vi "Get Color.vi"() -> (0 "Matched Color Name":string)   [LabVIEW 2019]
uses:
  Robot Global Data.vi
panel:
  out "Measured Color":cluster{"R":dbl, "G":dbl, "B":dbl}
  in  "Blue Calibration":cluster{"R":dbl, "G":dbl, "B":dbl}={"R"=0.143, "G"=0.427, "B"=0.429}
  in  "Green Calibration":cluster{"R":dbl, "G":dbl, "B":dbl}={"R"=0.197, "G"=0.561, "B"=0.24}
  in  "Red Calibration":cluster{"R":dbl, "G":dbl, "B":dbl}={"R"=0.561, "G"=0.323, "B"=0.114}
  in  "Yellow Calibration":cluster{"R":dbl, "G":dbl, "B":dbl}={"R"=0.361, "G"=0.524, "B"=0.113}
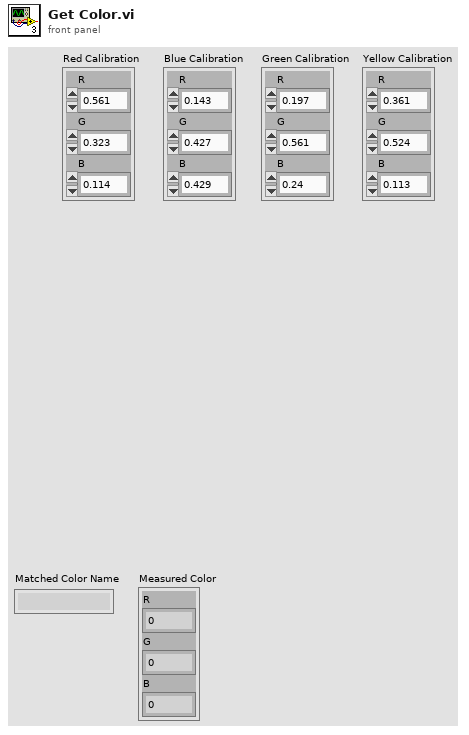
[diagram p1: front panel]
types:
  T1 = typedef "Color Sensor V3 DevRef.ctl" = cluster{"I2CDevRef":T2}
  T2 = typedef "WPI_I2CDevRef.ctl" = cluster{"DevStatus":errorcluster, "Device Address":u8, "Handle":i32, "I2C Bus":T3}
  T3 = typedef "i2c_bus.ctl" = enum16{"I2C On-Board", "I2C MXP", "Invalid"}
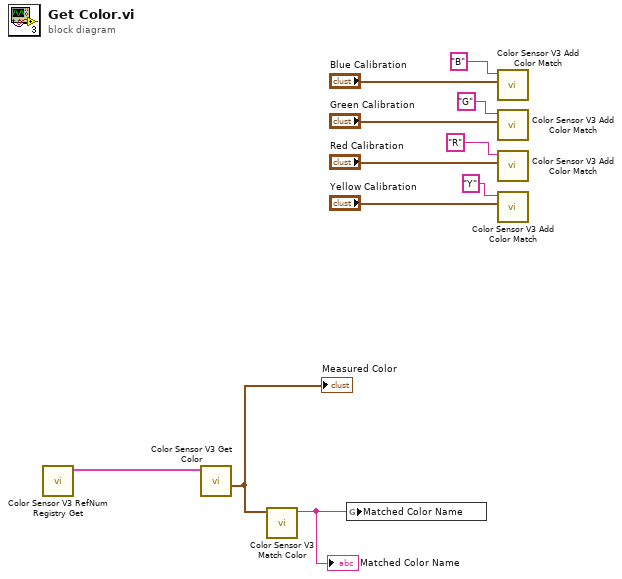
[diagram p0: block diagram]
diagram:
  n1 = call <vilib>:"Color Sensor V3 RefNum Registry Get.vi"() -> ("ColorSensorDevRef"=w2:T1)  [unwired: 10 in, 1 out]
  n2 = call <vilib>:"Color Sensor V3 Get Color.vi"("ColorSensorDevRef"=w2) -> ("Normalized Color"=w3:cluster{"R":dbl, "G":dbl, "B":dbl})  [unwired: 7 in, 3 out]
  "Measured Color" <- w3
  n3 = call <vilib>:"Color Sensor V3 Match Color.vi"("Measured Color"=w3) -> ("Matched Color Name"=w1:string)  [unwired: 8 in, 2 out]
  "Matched Color Name" <- w1
  n4 = global write "Robot Global Data.vi" "Matched Color Name"(w1) -> ()
  n5 = call <vilib>:"Color Sensor V3 Add Color Match.vi"("Color"="Blue Calibration", "Name"="B") -> ()  [unwired: 10 in]
  n6 = call <vilib>:"Color Sensor V3 Add Color Match.vi"("Color"="Green Calibration", "Name"="G") -> ()  [unwired: 10 in]
  n7 = call <vilib>:"Color Sensor V3 Add Color Match.vi"("Color"="Red Calibration", "Name"="R") -> ()  [unwired: 10 in]
  n8 = call <vilib>:"Color Sensor V3 Add Color Match.vi"("Color"="Yellow Calibration", "Name"="Y") -> ()  [unwired: 10 in]
